vi "Run Tests - When Tests Provided - Returns Same Amount Of Results.vi"(10 "Expected Amount":i32=-1, 11 "Test Cases":refnum<class "LVUnit Test Case.lvclass">[](array[class])) -> (0 "error out":errorcluster)   [LabVIEW 2017, in "LVUnit Test Executor.Tests.lvlib"]
uses:
  LVUnit Test Executor.Tests.lvlib
  LVUnit Test Case/LVUnit Test Case.lvclass
  C:/Users/pasca/Projects/Home/lvunit/Test Case/Test Case.lvclass
  LVUnit Test Executor/LVUnit Test Executor.lvclass
  <vilib>/PNR/Transparent Assertions/Transparent Assertions/Assertions/Assertions.lvlib
  Test Result/Test Result.lvclass
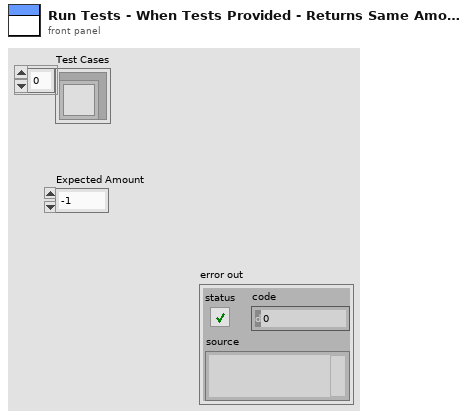
[diagram p1: front panel]
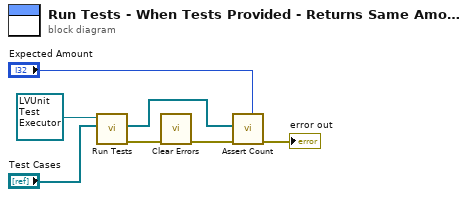
[diagram p0: block diagram]
diagram:
  n1 = call-dynamic "Run Tests.vi"("Test Cases"="Test Cases", "LVUnit Test Executor in"=refnum<class "LVUnit Test Executor.lvclass"> refnum ("LVUnit Test Executor")) -> ("error out"=w5:errorcluster, "Test Results"=w4:refnum<class "Test Result.lvclass">[])  [unwired: 7 in, 1 out]
  n2 = call <vilib>:"Clear Errors.vi"("error in (no error)"=w5) -> ("error out"=w1:errorcluster)  [unwired: 5 in, 1 out]
  n3 = call <vilib>:"Assert Count.vi"("Expected"="Expected Amount", "error in (no error)"=w1, "Haystack"=w4) -> ("error out"=→"error out":errorcluster)  [unwired: 8 in]
